vi "Choreo_DifferentialSample_ModuleForcesY.vi"(11 "ChoreoDifferentialSample":T1={"timestamp"=-999.0, "x"=0.0, "y"=0.0, "heading"=0.0, "velocityL"=0.0, "velocityR"=0.0, "angularVelocity"=0.0, "accelL"=0.0, "accelR"=0.0, "accelAngular"=0.0, "forceL"=0.0, "forceR"=0.0}) -> (3 "ForceR":dbl)   [LabVIEW 2019, in "ChoreoLib.lvlib"]
doc: "Retrieves the Right from a Differential Trajectory Sample\n\nInputs: \n -- ChoreoDifferentialSample - cluster - Differential sample.\n\nOutputs:\n -- ForceR - double - The force on Right wheel."
uses:
  ChoreoLib.lvlib
  TypeDef/ChoreoDifferentialSample.ctl
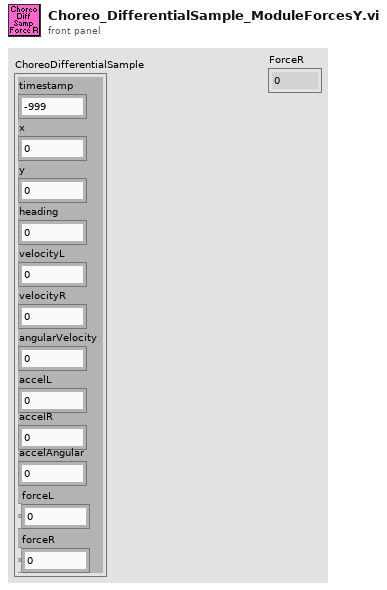
[diagram p1: front panel]
types:
  T1 = typedef "ChoreoLib.lvlib/ChoreoDifferentialSample.ctl" = cluster{"timestamp":dbl, "x":dbl, "y":dbl, "heading":dbl, "velocityL":dbl, "velocityR":dbl, "angularVelocity":dbl, "accelL":dbl, "accelR":dbl, "accelAngular":dbl, "forceL":dbl, "forceR":dbl}
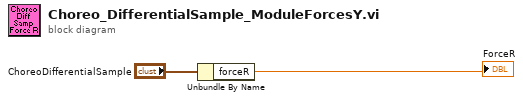
[diagram p0: block diagram]
diagram:
  n1 = Unbundle By Name("ChoreoDifferentialSample") -> ("forceR"=→"ForceR":dbl)
